vi "Tx_Rx.vi"(4 "Wait for? (\\n)":string="\n", 6 "TermChar (\\n)":string="\n", 7 "Timeout (3000)":i32=3000, 8 "error in":errorcluster, 9 "Write":string, 10 "Fbk? (T)":bool=TRUE, 11 "VISA in":refnum<visa-resource-name>) -> (0 "error out":errorcluster, 1 "Read":string, 2 "Timeout?":bool, 3 "VISA out":refnum<visa-resource-name>, 5 "ExecTime (ms)":i32)   [LabVIEW 2016, in "Serial_G.lvlib"]
doc: "Sends a command and recieves cmd response if \"Fbk\" set to T"
uses:
  Serial_G.lvlib
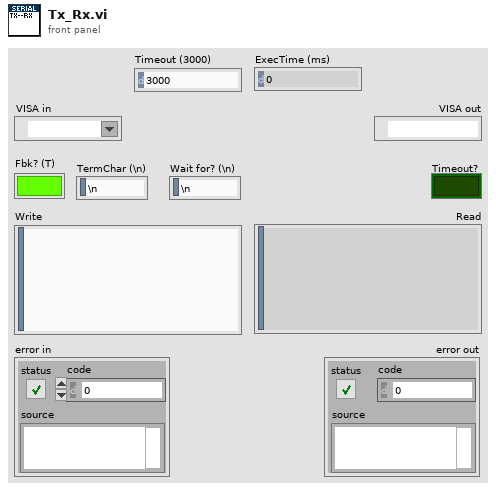
[diagram p1: front panel]
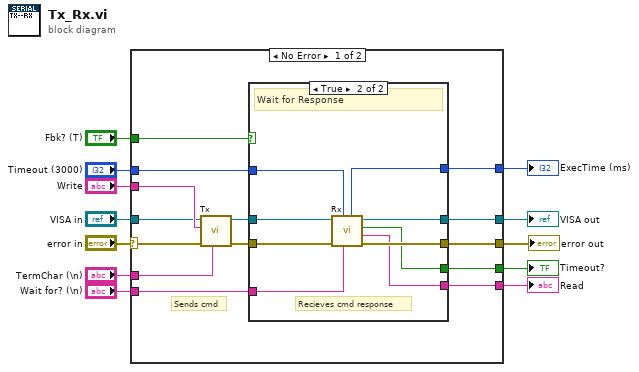
[diagram p0: block diagram]
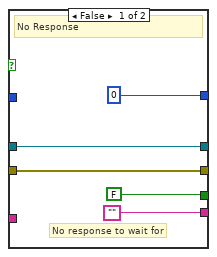
[diagram p2: hidden frame]
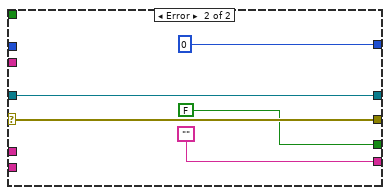
[diagram p3: hidden frame]
diagram:
  n1 = case shown="No Error" "error in" {
    selector: "error in" -> [w13 w45]
    tunnel: [w24 w45] -> w11
    tunnel: "Fbk? (T)" -> [w23 _]
    tunnel: "Timeout (3000)" -> [w22 _]
    tunnel: "Write" -> [w21 _]
    tunnel: "TermChar (\\n)" -> [w14 _]
    tunnel: "VISA in" -> [w20 w43]
    tunnel: "Wait for? (\\n)" -> [w19 _]
    tunnel: [w18 0 ("ExecTime(ms)")] -> w4
    tunnel: [w17 w43] -> w3
    tunnel: [w16 FALSE ("Timeout?")] -> w2
    tunnel: [w15 "" ("Response")] -> w1
    frame No Error {
      # "Sends cmd"
      n2 = call "Tx.vi"("TermChar (\\r\\n)"=w14, "error in"=w13, "Command"=w21, "VISA in"=w20) -> ("error out"=w25:errorcluster, "VISA out"=w26:refnum<visa-resource-name>)  [unwired: 6 in]
      n3 = case shown="True" w23 {
        tunnel: w26 -> [w31 w40]
        tunnel: w25 -> [w29 w39]
        tunnel: w22 -> [_ w36]
        tunnel: [w29 w38] -> w24
        tunnel: [0 ("Time (ms)") w35] -> w18
        tunnel: w19 -> [_ w32]
        tunnel: [w31 w37] -> w17
        tunnel: [FALSE ("Timeout?") w34] -> w16
        tunnel: ["" w33] -> w15
        frame False {
          # "No response to wait for"
          # "No Response"
        }
        frame True {
          # "Recieves cmd response"
          # "Wait for Response"
          n4 = call "Rx.vi"("Wait for? (\\r\\n)"=w32, "Timeout_ms (3000)"=w36, "error in"=w39, "VISA in"=w40) -> ("error out"=w38:errorcluster, "Response"=w33:string, "Timeout?"=w34:bool, "VISA out"=w37:refnum<visa-resource-name>, "ExecTime(ms)"=w35:i32)  [unwired: 3 in]
        }
      }
    }
    frame Error {
    }
  }
  "error out" <- w11
  "Read" <- w1
  "VISA out" <- w3
  "Timeout?" <- w2
  "ExecTime (ms)" <- w4
